vi "cluster_ccd_status.vi"() -> ()   [LabVIEW 2018]
panel:
  out "Camera Status":T1
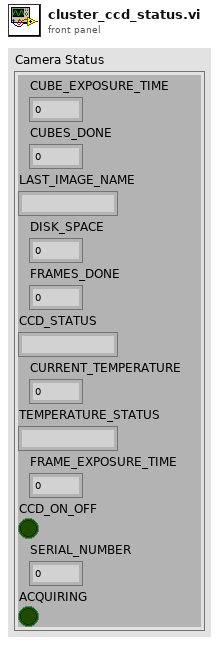
[diagram p1: front panel]
types:
  T1 = cluster{"CUBE_EXPOSURE_TIME":sgl, "CUBES_DONE":u16, "LAST_IMAGE_NAME":string, "DISK_SPACE":u16, "FRAMES_DONE":u16, "CCD_STATUS":string, "CURRENT_TEMPERATURE":i16, "TEMPERATURE_STATUS":string, "FRAME_EXPOSURE_TIME":u16, "CCD_ON_OFF":bool, "SERIAL_NUMBER":u16, "ACQUIRING":bool}
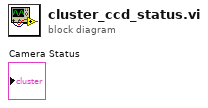
[diagram p0: block diagram]
diagram:
